vi "SigGen-Compute Max Level (AdvFilt).vi"(0 "Waveform":T21(xcontrol), 5 "Filter XCtl":T4(xcontrol), 9 "Level":T1, 11 "error in (no error)":errorcluster, 12 "Sampling Rate (Hz)":dbl, 13 "Npts":i32) -> (10 "Level out":T1, 14 "Max Level":dbl, 15 "error out":errorcluster)   [LabVIEW 2015]
uses:
  Controls/Waveform XCtl/Waveform XCtl.xctl
  Controls/Advanced Filter XCtl/Advanced Filter XCtl.xctl
  Controls/Level XCtl/Level Data.ctl
  Controls/Level XCtl/Level Units.ctl
  Controls/Level XCtl/Level XCtl.xctl
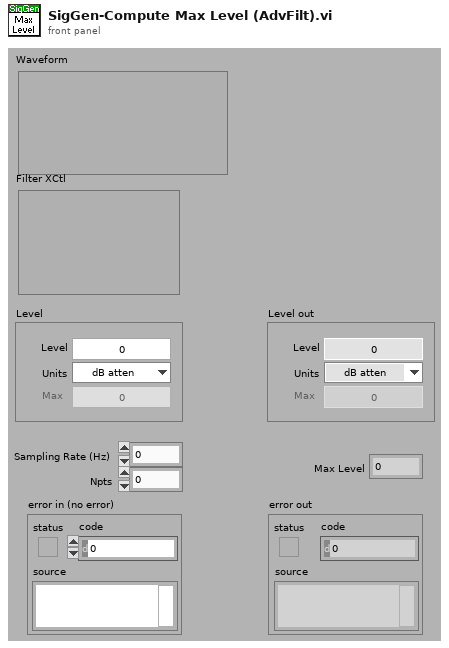
[diagram p1: front panel]
types:
  T1 = typedef "Level XCtl.xctl/Level Data.ctl" = cluster{"Level":dbl, "Units":T2, "Max":dbl, "Multiplier":dbl, "Cal File":path, "Cal":cluster{"Freq (Hz)":dbl[], "Mag (dB SPL)":dbl[], "Phase (deg)":dbl[]}}
  T2 = typedef "Level Units.ctl" = enum16{"dB atten", "dB SPL", "dB re 1 Vrms", "dB V/Hz½", "mW", "dB HL", "Volts", "dB mW"}
  T3 = typedef "Filter-Bandwidth Units.ctl" = enum16{"Linear", "Octaves", "Min-Max"}
  T4 = cluster{"Type":enum16{"Lowpass", "Highpass", "Bandpass", "Bandstop", "OFF"}, "CF (kHz)":dbl, "BW (kHz)":dbl, "Cascade":bool, "Quadrature":bool, "Scale Factor":dbl, "Stages":cluster{"IIR Filter":cluster{"filter structure":enum32{"IIR 2nd Order", "IIR 4th Order"}, "Reverse Coefficients":dbl[], "Forward Coefficients":dbl[]}, "State":dbl[]}[], "Class":enum16{"Elliptic", "Butterworth"}, "Order":i32, "BWUnits":T3}
  T5 = typedef "Waveform Enum.ctl" = enum16{"OFF", "Tone", "Noise", "Pulse Train", "File", "FM Sweep", "Chirp Train", "Complex Tone", "FM Tone", "Moving Ripple"}
  T6 = typedef "Tone Params.ctl" = cluster{"Frequency (kHz)":dbl, "Last Freq":dbl, "Last Phase":dbl}
  T7 = typedef "Pulse Train Params.ctl" = cluster{"Pulse width (us)":dbl, "Pulse rate (Hz)":dbl, "Gap (ms)":dbl, "Polarity":T8, "PT State":T9, "Asynch":bool}
  T8 = typedef "Pulse Polarity.ctl" = enum16{"POS", "NEG", "POS-NEG", "NEG-POS"}
  T9 = typedef "PT-Continuous State.ctl" = cluster{"Template":dbl[], "Nperiod":i32, "Index":i32, "Pulse Rate (Hz)":dbl, "Phase (cycles)":dbl, "Noff":i32}
  T10 = typedef "Noise Params.ctl" = cluster{"InvFilt":bool, "Noise":dbl[], "CurPt":i32, "Aweight":bool, "Seed":i32, "afile":path}
  T11 = typedef "StimFile-Params.ctl" = cluster{"Filename":path, "Signal":dbl[], "Channel":i32, "stream":bool, "offset":i32, "nreps":i32, "loops":i32}
  T12 = typedef "FM Sweep Params.ctl" = cluster{"Rate (oct/s)":dbl, "Fmin (Hz)":dbl, "Fmax (Hz)":dbl, "Ramp (ms)":dbl, "Linear":bool}
  T13 = typedef "Chirp Train.ctl" = cluster{"Params":T14, "Data":cluster{"WF":dbl[]}}
  T14 = typedef "Chirp Train Params.ctl" = cluster{"Fmin (kHz)":dbl, "Fmax (kHz)":dbl, "Compensate":bool, "Duration (ms)":dbl}
  T15 = typedef "CT-Params.ctl" = cluster{"F0 (Hz)":dbl, "Band":cluster{"Flow (Hz)":dbl, "Fhigh (Hz)":dbl}, "Phase":T16, "Min F0 (Hz)":dbl, "Max F0 (Hz)":dbl, "ContinRandPhase":bool, "Max peak factor":dbl, "Max mod depth":dbl, "MinHarmNum":i32, "MaxHarmNum":i32, "Level Mode":enum16{"per component", "overall rms"}, "% jitter":dbl}
  T16 = typedef "CT-Phase Enum.ctl" = enum16{"Cosine", "Random", "Alternating"}
  T17 = typedef "CT-Runtime Data.ctl" = cluster{"Ncomp":i32, "MinHarm":i32, "Phase":dbl[], "Amplitude":dbl[], "Npts/frame":i32, "Last F0":dbl, "Fmin":dbl, "Fmax":dbl, "Lslope":dbl, "randphase":bool, "overall rms":bool, "fmult":dbl[], "jittered":bool}
  T18 = typedef "Moving Ripple.ctl" = cluster{"Params":T19, "Data":T20}
  T19 = typedef "Moving Ripple.Params.ctl" = cluster{"Fmin":dbl, "Fmax":dbl, "Density":dbl, "Velocity":dbl, "Depth":dbl, "Phase":dbl, "Comp/oct":i32}
  T20 = typedef "Moving Ripple.Data.ctl" = cluster{"Freq":dbl[], "A":dbl[], "phase":dbl[], "Phase":dbl}
  T21 = cluster{"Type":T5, "Tone":T6, "Pulse Train":T7, "Noise":T10, "File":T11, "FMSweep":T12, "Chirp Train":T13, "Complex Tone":cluster{"Params":T15, "Data":T17}, "Moving Ripple":T18}
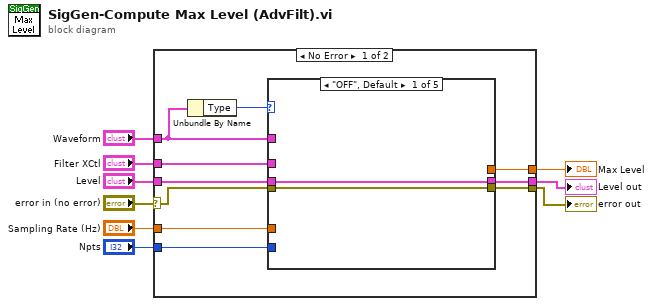
[diagram p0: block diagram]
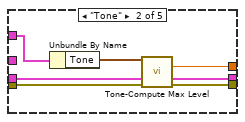
[diagram p2: hidden frame]
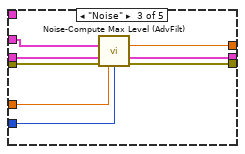
[diagram p3: hidden frame]
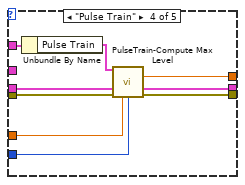
[diagram p4: hidden frame]
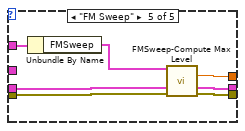
[diagram p5: hidden frame]
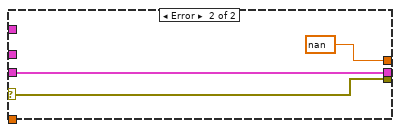
[diagram p6: hidden frame]
diagram:
  n1 = case shown="No Error" "error in (no error)" {
    selector: "error in (no error)" -> [w17 w55]
    tunnel: "Level" -> [w16 w53]
    tunnel: "Waveform" -> [w18 _]
    tunnel: "Filter XCtl" -> [w13 _]
    tunnel: [w11 w55] -> w8
    tunnel: "Npts" -> [w14 _]
    tunnel: [w10 nan ("Reference Level")] -> w3
    tunnel: "Sampling Rate (Hz)" -> [w15 _]
    tunnel: [w12 w53] -> w1
    frame No Error {
      n2 = Unbundle By Name(w18) -> ("Type"=w19:T5)
      n3 = case shown="\"OFF\", Default" w19 {
        tunnel: w18 -> [_ w28 _ w45 w52]
        tunnel: w17 -> [w20 w26 w36 w40 w50]
        tunnel: w16 -> [w21 w25 w35 w39 w48]
        tunnel: w15 -> [_ _ w34 w38 _]
        tunnel: w14 -> [_ _ w33 w37 _]
        tunnel: w13 -> [_ _ w29 _ _]
        tunnel: [w21 w23 w31 w42 w47] -> w12
        tunnel: [w20 w24 w30 w41 w49] -> w11
        tunnel: [_ w22 w32 w43 w46] -> w10
        frame "OFF", Default {
        }
        frame "Tone" {
          n4 = Unbundle By Name(w28) -> ("Tone"=w27:T6)
          n5 = call "Tone-Compute Max Level.vi"("Tone Params"=w27, "Level"=w25, "error in (no error)"=w26) -> ("Max Level"=w22:dbl, "Level out"=w23:T1, "error out"=w24:errorcluster)  [unwired: 10 in]
        }
        frame "Noise" {
          n6 = call "Noise-Compute Max Level (AdvFilt).vi"("Filter XCtl"=w29, "Level"=w35, "error in (no error)"=w36, "Sampling Rate (Hz)"=w34, "Npts"=w33) -> ("Max Level"=w32:dbl, "Level out"=w31:T1, "error out"=w30:errorcluster)  [unwired: 8 in]
        }
        frame "Pulse Train" {
          n7 = Unbundle By Name(w45) -> ("Pulse Train"=w44:T7)
          n8 = call "PulseTrain-Compute Max Level.vi"("Pulse Train Params"=w44, "Level"=w39, "error in (no error)"=w40, "Sampling Rate (Hz)"=w38, "Npts"=w37) -> ("Max Level"=w43:dbl, "Level out"=w42:T1, "error out"=w41:errorcluster)  [unwired: 8 in]
        }
        frame "FM Sweep" {
          n9 = Unbundle By Name(w52) -> ("FMSweep"=w51:T12)
          n10 = call "FMSweep-Compute Max Level.vi"("FMSweep"=w51, "Level"=w48, "error in (no error)"=w50) -> ("Max Level"=w46:dbl, "Level out"=w47:T1, "error out"=w49:errorcluster)  [unwired: 10 in]
        }
      }
    }
    frame Error {
    }
  }
  "error out" <- w8
  "Max Level" <- w3
  "Level out" <- w1
